vi "Read ModeArray.vi"(8 "error in (no error)":errorcluster, 11 "ModeCol in":refnum<class "ModeCol.lvclass">) -> (0 "error out":errorcluster, 2 "Array":T1(array[cluster])=[{"Mode"="Continue", "ModeTag"="MODE_CONTINUE", "Disables?"=TRUE}, {"Mode"="Ramp", "ModeTag"="MODE_RAMP", "Disables?"=FALSE}, {"Mode"="Loop", "ModeTag"="MODE_LOOP", "Disables?"=TRUE}, {"Mode"="EndLoop", "ModeTag"="MODE_ENDLOOP", "Disables?"=TRUE}], 3 "ModeCol out":refnum<class "ModeCol.lvclass">)   [LabVIEW 2013, in "ModeCol.lvclass"]
uses:
  ModeCol.lvclass
  ModeCol.lvclass/ModeCol.ctl
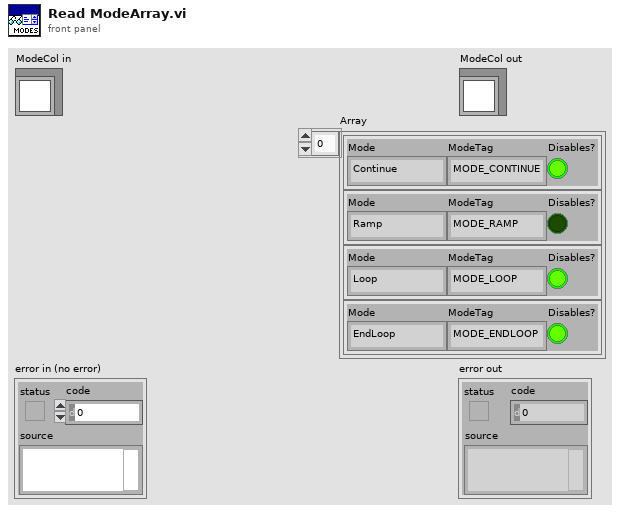
[diagram p1: front panel]
types:
  T1 = cluster{"Mode":string, "ModeTag":string, "Disables?":bool}[]
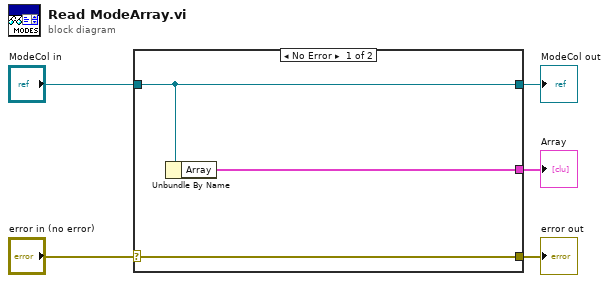
[diagram p0: block diagram]
diagram:
  n1 = case shown="No Error" "error in (no error)" {
    selector: "error in (no error)" -> [w8 w9]
    tunnel: [w8 w9] -> w4
    tunnel: [w7 w10] -> w2
    tunnel: "ModeCol in" -> [w7 w10]
    tunnel: [w6 _] -> w1
    frame No Error {
      n2 = Unbundle By Name(w7) -> ("Array"=w6:T1)
    }
    frame Error {
    }
  }
  "error out" <- w4
  "ModeCol out" <- w2
  "Array" <- w1
